vi "Add Custom Device.vi"(7 "Overwrite Existing?":bool=TRUE, 8 "error in (no error)":errorcluster, 9 "Settings":T1, 10 "Base Node Path":string, 11 "SysDef Ref":T2) -> (0 "error out":errorcluster, 2 "New Node Path":string, 3 "SysDef Ref Out":T2)   [LabVIEW 2019, in "Simple SysDef API.lvlib"]
uses:
  <userlib>/SimpleSysDef/Simple SysDef API.lvlib
  <userlib>/SimpleSysDef/_SubVIs/System Definition Reference.ctl
  NationalInstruments.VeriStand.SystemDefinitionAPI
  <userlib>/SimpleSysDef/_SubVIs/Add Custom Device_Settings.ctl
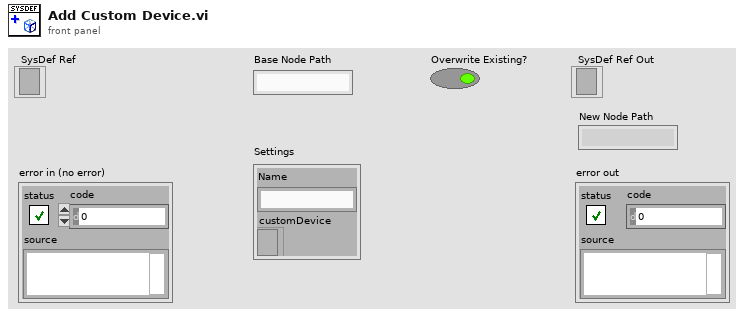
[diagram p1: front panel]
types:
  T1 = typedef "Simple SysDef API.lvlib/Add Custom Device_Settings.ctl" = cluster{"Name":string, "customDevice":refnum<k24>}
  T2 = typedef "Simple SysDef API.lvlib/System Definition Reference.ctl" = refnum<k24>
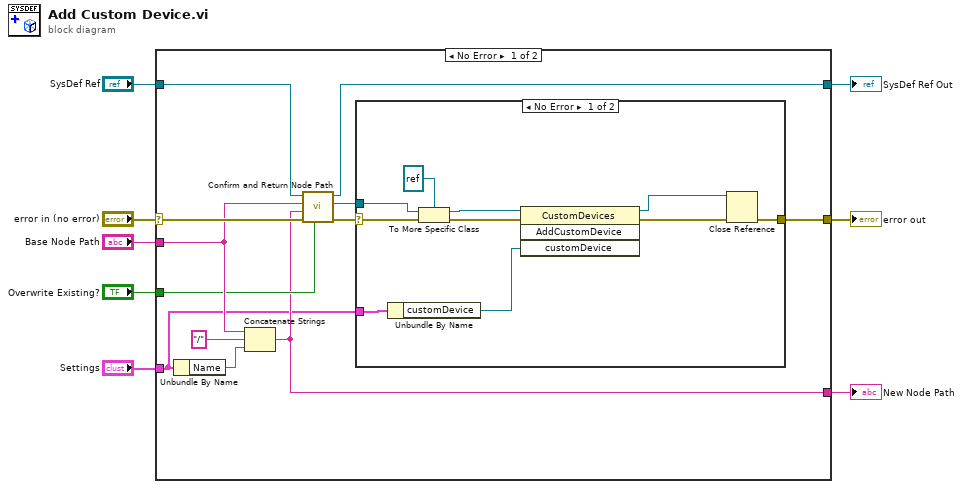
[diagram p0: block diagram]
diagram:
  n1 = case shown="No Error" "error in (no error)" {
    selector: "error in (no error)" -> [w20 w33]
    tunnel: [w15 w33] -> w7
    tunnel: "SysDef Ref" -> [w19 w32]
    tunnel: [w18 w32] -> w5
    tunnel: "Base Node Path" -> [w12 _]
    tunnel: "Overwrite Existing?" -> [w11 _]
    tunnel: "Settings" -> [w9 _]
    tunnel: [w10 _] -> w1
    frame No Error {
      n2 = Unbundle By Name(w9) -> ("Name"=w16:string)
      n3 = Concatenate Strings(w12, "/" ("string"), w16) -> (w10:string)
      n4 = call <userlib>:"Confirm and Return Node Path.vi"("Overwrite Existing?"=w11, "error in (no error)"=w20, "New Node Path"=w10, "Base Node Path"=w12, "SysDef Ref"=w19) -> ("error out"=w13:errorcluster, "Node Ref"=w14:refnum<k24>, "SysDef Ref Out"=w18:T2)  [unwired: 4 in]
      n5 = case shown="No Error" w13 {
        selector: w13 -> [w29 w31]
        tunnel: [w28 w31] -> w15
        tunnel: w14 -> [w30 _]
        tunnel: w9 -> [w22 _]
        frame No Error {
          n6 = Unbundle By Name(w22) -> ("customDevice"=w21:refnum<k24>)
          n7 = To More Specific Class(target class=refnum<k24> refnum ("Node Ref"), reference=w30, error in=w29) -> (specific class reference=w26:refnum<k24>, error out=w25:errorcluster)
          n8 = invoke class="CustomDevices" method="AddCustomDevice"(reference=w26, error in=w25, "customDevice"=w21) -> (reference out=w23:refnum<k24>, error out=w24:errorcluster)  [unwired: 1 in, 2 out]
          n9 = Close Reference(reference=w23, error in (no error)=w24) -> (error out=w28:errorcluster)
        }
        frame Error {
        }
      }
    }
    frame Error {
    }
  }
  "SysDef Ref Out" <- w5
  "error out" <- w7
  "New Node Path" <- w1
